vi "Stepper_Sub_VI.vi"(6 "Numeric":dbl, 8 "Direction":bool, 9 "Numeric 2":i32, 10 "milliseconds to wait":u32) -> ()   [LabVIEW 2016]
uses:
  <vilib>/myRIO/Common/Instrument Driver Framework/myRIO v1.0/DIO/typedefs/DIO Channels Enum.ctl
  <vilib>/myRIO/Common/Instrument Driver Framework/myRIO v1.0/DIO/typedefs/DIO Channels List.ctl
  <vilib>/myRIO/Common/Instrument Driver Framework/Utilities/typedefs/Generic FPGA Reference.ctl
  <vilib>/myRIO/Common/Instrument Driver Framework/Utilities/typedefs/myRIO v1.0 Reference.ctl
  <vilib>/myRIO/Common/Instrument Driver Framework/Utilities/typedefs/Hardware Version Enum.ctl
  <vilib>/myRIO/Common/Instrument Driver Framework/Utilities/typedefs/myRIO Generic Hardware Reference.ctl
  <vilib>/myRIO/Instrument Drivers/Onboard IO/DIO/typedefs/DIO Reference.ctl
  <vilib>/myRIO/Instrument Drivers/Onboard IO/DIO/DIO.lvlib
  <vilib>/myRIO/Instrument Drivers/Onboard IO/DIO/vis/Write.vi
  <vilib>/userdefined/High Color/nirio_resource_hc.ctl
  <vilib>/myRIO/Common/Instrument Driver Framework/myRIO v1.0/DIO/vis/myRIO v1.1 Open DIO.vi
  <vilib>/myRIO/Instrument Drivers/Onboard IO/DIO/vis/myRIO DIO Open.xnode
  <vilib>/myRIO/Common/Instrument Driver Framework/Utilities/vis/Is FPGA Ref Available.vi
  <vilib>/myRIO/Express VI/Onboard IO/DO/DO Express VI.xnode
  <vilib>/myRIO/Express VI/Onboard Devices/LED/LED Express VI.xnode
panel:
  out "Boolean":bool
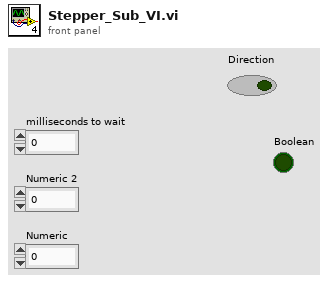
[diagram p1: front panel]
types:
  T1 = typedef "DIO.lvlib/DIO Reference.ctl" = cluster{"myRIO Reference":T2, "DIO Channels List":T6}
  T2 = typedef "myRIO Generic Hardware Reference.ctl" = cluster{"myRIO Model":T3, "myRIO Hardware Reference":T4}
  T3 = typedef "Hardware Version Enum.ctl" = enum16{"Unknown", "myRIO-1900", "myRIO-1950", "roboRIO", "NI ELVIS RIO CM"}
  T4 = typedef "myRIO v1.0 Reference.ctl" = cluster{"Generic FPGA Reference":T5, "Allow multiple opens":bool}
  T5 = typedef "Generic FPGA Reference.ctl" = refnum<k20>
  T6 = typedef "DIO Channels List.ctl" = T7[]
  T7 = typedef "DIO Channels Enum.ctl" = enum16{"Not Connected", "C/DIO0", "C/DIO1", "C/DIO2", "C/DIO3", "C/DIO4", "C/DIO5", "C/DIO6", "C/DIO7", "A/DIO0", "A/DIO1", "A/DIO2", "A/DIO3", "A/DIO4", "A/DIO5", "A/DIO6", "A/DIO7", "A/DIO8", "A/DIO9", "A/DIO10", "A/DIO11", "A/DIO12", "A/DIO13", "A/DIO14", "A/DIO15", "B/DIO0", "B/DIO1", "B/DIO2", "B/DIO3", "B/DIO4", "B/DIO5", "B/DIO6", "B/DIO7", "B/DIO8", "B/DIO9", "B/DIO10", "B/DIO11", "B/DIO12", "B/DIO13", "B/DIO14", "B/DIO15", "LED0", "LED1", "LED2", "LED3", "Button0", "DIO/DIO0", "DIO/DIO1", "DIO/DIO2", "DIO/DIO3", "DIO/DIO4", "DIO/DIO5", "DIO/DIO6", "DIO/DIO7", "DIO/DIO8", "DIO/DIO9", "SPI/CS0", "SPI/CS1", "SPI/CS2", "SPI/CS3", "LED RADIO (Green)", "LED RADIO (Red)", "LED COMM (Green)", "LED COMM (Red)", "LED MODE (Green)", "LED MODE (Red)"}
  T8 = typedef "nirio_resource_hc.ctl" = tag
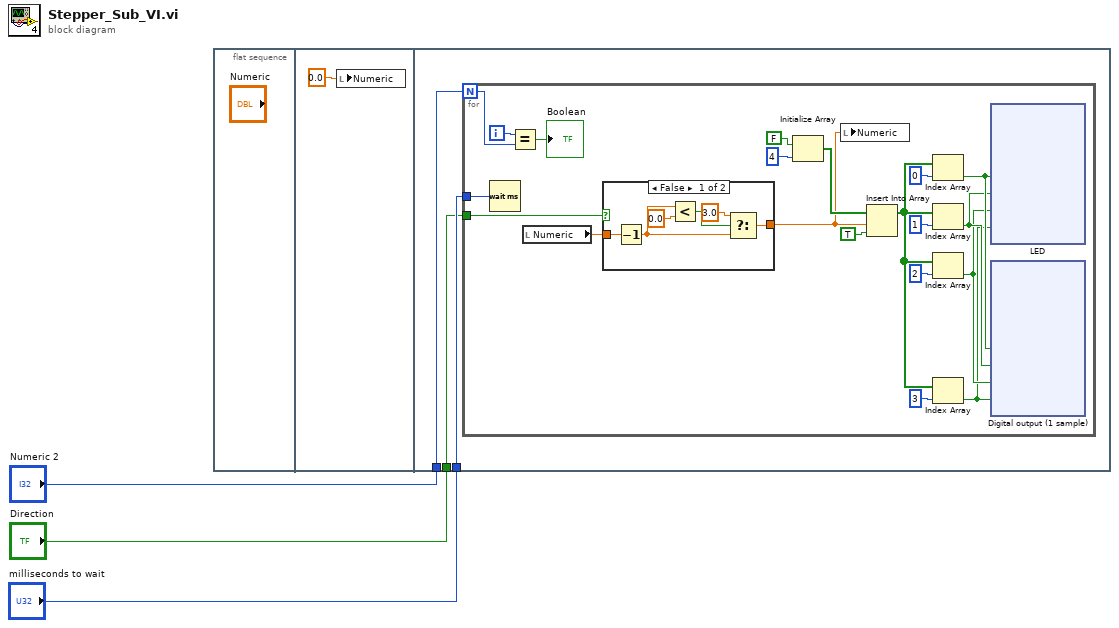
[diagram p0: block diagram]
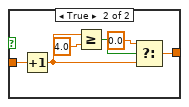
[diagram p2: hidden frame]
diagram:
  n1 = flat-sequence {
    tunnel: "Numeric 2" -> [w7]
    tunnel: "milliseconds to wait" -> [w6]
    tunnel: "Direction" -> [w5]
    frame #0 {
    }
    frame #1 {
      n2 = local write "Numeric"(0.0 ("Numeric")) -> ()
    }
    frame #2 {
      n3 = for {
        N: w7 -> [w9]
        tunnel: w6 -> [w27]
        tunnel: w5 -> [w17]
        i -> [w10]
        n4 = Wait (ms)(milliseconds to wait=w27) -> ()  [unwired: 1 out]
        n5 = Equal?(x=w10, y=w9) -> (x = y?=→"Boolean":bool)
        n6 = local read "Numeric"() -> (w16:dbl)
        n7 = case shown="False" w17 {
          tunnel: w16 -> [w67 w73]
          tunnel: [w68 w72] -> w15
          frame False {
            n8 = Decrement(x=w67) -> (x-1=w66:dbl)
            n9 = Less?(x=w66, y=0.0) -> (x < y?=w69:bool)
            n10 = Select(t=3.0, s=w69, f=w66) -> (s? t:f=w68:dbl)
          }
          frame True {
            n11 = Increment(x=w73) -> (x+1=w74:dbl)
            n12 = Greater Or Equal?(x=w74, y=4.0) -> (x >= y?=w75:bool)
            n13 = Select(t=0.0, s=w75, f=w74) -> (s? t:f=w72:dbl)
          }
        }
        n14 = Initialize Array(FALSE, 4 ("dimension size")) -> (w24:bool[])
        n15 = local write "Numeric"(w15) -> ()
        n16 = Insert Into Array(array=w24, index=w15, new element=TRUE) -> (w18:bool[])
        n17 = Index Array(array=w18, index=0) -> (element=w14:bool)
        n18 = Index Array(array=w18, index=1) -> (element=w13:bool)
        n19 = Index Array(array=w18, index=2) -> (element=w12:bool)
        n20 = Index Array(array=w18, index=3) -> (element=w11:bool)
        n21 = xnode "LED"("LED0"=w14, "LED1"=w13, "LED2"=w12, "LED3"=w11) -> ()  [unwired: 1 in, 1 out]
        n22 = xnode "Digital output (1 sample)"("IN4 (A/DIO10 (Pin 31))"=w14, "IN3 (A/DIO11 (Pin 18))"=w13, "IN2 (A/DIO13 (Pin 26))"=w12, "IN1 (A/DIO15 (Pin 34))"=w11) -> ()  [unwired: 1 in, 1 out]
      }
    }
  }
